vi "CSM - Make String Arguments Safe.vi"(2 "Argument String":string="eaasdf->fqwvrf", 4 "Ignore Argument Type(F)":bool) -> (7 "Safe Argument String":string)   [LabVIEW 2017, in "Communicable State Machine.lvlib"]
doc: "Converts CSM keywords in the argument string to %Hex format to ensure that CSM message string parsing is not affected.\n\n\n> [!NOTE] <b>CSM Message Keywords</b>\n>\n> The following are CSM message keywords: `->`, `->|`, `-@`, `-&`, `<-`, `\\r`, `\\n`, `//`, `>>`, `>>>`, `>>>>`, `;`, `,`.\n\n\n> [!NOTE] <b>CSM Safe String Argument</b>\n>\n> To pass arbitrary strings in CSM arguments without disrupting message parsing, CSM has a built-in Safe-String encoding/decoding scheme. The argument type string is SAFESTR. The conversion process is as follows:\n> 1. Replace `%` in the input string with `%25`.\n> 2. Scan the string. If any CSM keywords, such as `->`, `;`, `\\r` appear, replace them with `%Hex` escape sequences.\n> 3. Obtain the argument in the form `<SAFESTR> escaped string`, which can be safely embedded in the state string without disrupting CSM message parsing.\n> Decoding is the reverse process: the `%Hex` escape sequences of CSM keywords are converted back first, then `%25` is converted back to `%`.\n\n\n<b>Reference Example</b>: `[CSM-Example]\\0. Base Concepts\\4.3 Arguments - Safe Arguments if it contains key words of CSM.vi`.\n\n-- <b>Controls</b> --\n- <b>Argument String</b>: String argument.\n- <b>Ignore Argument Type(F)</b>: Do not append argument type `SAFESTR`.\n\n-- <b>Indicators</b> --\n- <b>Safe Argument String</b>: Safe string argument."
uses:
  Communicable State Machine.lvlib
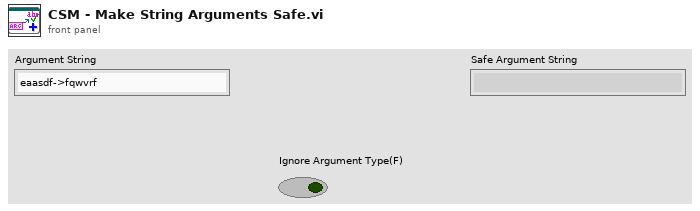
[diagram p1: front panel]
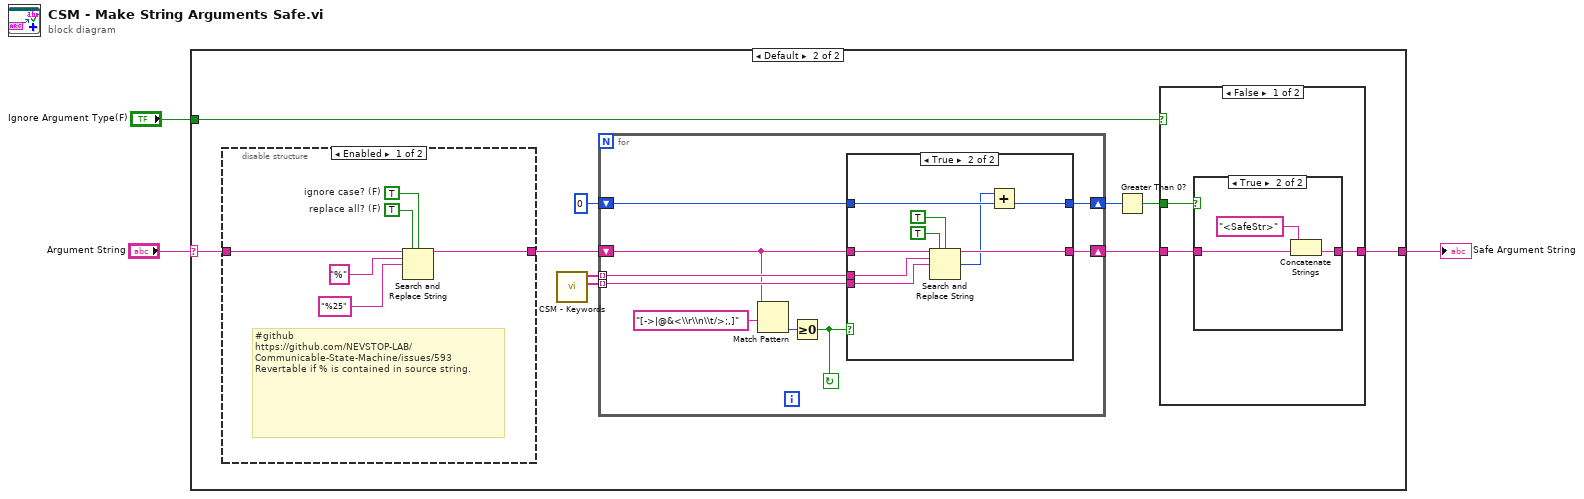
[diagram p0: block diagram]
diagram:
  n1 = case shown="Default" "Argument String" {
    selector: "Argument String" -> [_ w4]
    tunnel: [_ w13] -> w2
    tunnel: "Ignore Argument Type(F)" -> [_ w12]
    frame "" {
    }
    frame Default {
      n2 = disable-structure shown="Enabled" {
        disable-tunnel: [w19 w20] -> w5
        disable-tunnel: w4 -> [w18 w20]
        frame Enabled {
          w15 = TRUE  # ignore case? (F)
          w16 = TRUE  # replace all? (F)
          # "#github \nhttps://github.com/NEVSTOP-LAB/Communicable-State-Machine/issues/593\nRevertable if % is contained in source string."
          n3 = Search and Replace String(replace all?=w16, case sensitive?=w15, input string=w18, search string="%", replace string="%25" ("search string")) -> (result string=w19:string)  [unwired: 3 in, 3 out]
        }
        frame Disabled {
        }
      }
      n4 = call "CSM - Keywords.vi"() -> ("Keywords (%Hex Format)"=w10:string[], "Keywords"=w11:string[])  [unwired: 10 in]
      n5 = for {
        shift-right: [w37] -> w9
        shift-left: w5 -> [w30]
        tunnel: w10 -> [w35] mode=indexing
        tunnel: w11 -> [w36] mode=indexing
        shift-right: [w33] -> w7
        shift-left: 0 -> [w34]
        stop <- w29 continue-if-true
        n6 = Match Pattern(string=w30, regular expression="[->|@&<\\r\\n\\t/>;,]") -> (offset past match=w32:i32)  [unwired: 1 in, 3 out]
        n7 = Greater Or Equal To 0?(x=w32) -> (x >= 0?=w29:bool)
        n8 = case shown="True" w29 {
          tunnel: [w38 w47] -> w37
          tunnel: w36 -> [_ w46]
          tunnel: w35 -> [_ w45]
          tunnel: w34 -> [w39 w44]
          tunnel: [w39 w43] -> w33
          tunnel: w30 -> [w38 w41]
          frame False {
          }
          frame True {
            n9 = Search and Replace String(replace all?=TRUE ("replace all? (F)"), case sensitive?=TRUE ("ignore case? (F)"), input string=w41, search string=w46, replace string=w45) -> (result string=w47:string, number of replacements=w42:i32)  [unwired: 3 in, 2 out]
            n10 = Add(x=w42, y=w44) -> (x+y=w43:i32)
          }
        }
      }
      n11 = Greater Than 0?(x=w7) -> (x > 0?=w6:bool)
      n12 = case shown="False" w12 {
        tunnel: w9 -> [w23 w28]
        tunnel: [w22 w28] -> w13
        tunnel: w6 -> [w21 _]
        frame False {
          n13 = case shown="True" w21 {
            tunnel: w23 -> [w24 w26]
            tunnel: [w24 w25] -> w22
            frame False {
            }
            frame True {
              n14 = Concatenate Strings("<SafeStr>" ("string"), w26) -> (w25:string)
            }
          }
        }
        frame True {
        }
      }
    }
  }
  "Safe Argument String" <- w2
